vi "Binary to LEUI.vi"(7 "Numeric":u8) -> (8 "Blinking LED":T1)   [LabVIEW 2016, in "TLMB.lvlib"]
doc: "This VI converts a binary number to the expected display on LEUI"
uses:
  Projects/TLMB.lvlib
  controls/LEUI_LEDs.ctl
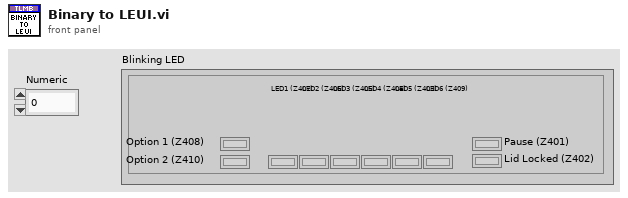
[diagram p1: front panel]
types:
  T1 = typedef "TLMB.lvlib/LEUI_LEDs.ctl" = cluster{"Pause (Z401)":bool, "Lid Locked (Z402)":bool, "LED1 (Z407)":bool, "LED2 (Z406)":bool, "LED3 (Z405)":bool, "LED4 (Z404)":bool, "LED5 (Z403)":bool, "LED6 (Z409)":bool, "Option 1 (Z408)":bool, "Option 2 (Z410)":bool}
  T2 = cluster{"[0]":bool, "[1]":bool, "[2]":bool, "[3]":bool, "[4]":bool, "[5]":bool, "[6]":bool, "[7]":bool, "[8]":bool, "[9]":bool}
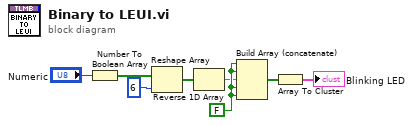
[diagram p0: block diagram]
diagram:
  w8 = FALSE
  n1 = Number To Boolean Array(number="Numeric") -> (Boolean array=w3:bool[])
  n2 = Reshape Array(w3, 6 ("dimension size")) -> (w2:bool[])
  n3 = Reverse 1D Array(array=w2) -> (reversed array=w4:bool[])
  n4 = Build Array (concatenate)(w8, w8, w4, w8, w8) -> (w6:bool[])
  n5 = Array To Cluster(array=w6) -> (cluster=→"Blinking LED":T2)
